vi "EESPY_Read.vi"(2 "I/O Voltage Level":i32(ring)=33 items=["3.3V"=33, "2.5V"=25, "1.8V"=18, "1.5V"=15, "1.2V"=12], 3 "Line Number":u8, 4 "device reference in":T2) -> (0 "Value":bool, 1 "Read Value":T1 items=["0 (Logic Low)", "1 (Logic High)"])   [LabVIEW 2016]
doc: "This basic DIO example uses the DIO basic API to read a digital line. It allows you to change the line number and I/O voltage.\n\nThe parameters will have the following effects:\nLine Number specifies the DIO line to read.\n\nThe I/O Voltage Level property configures the NI-845x reference voltage to the desired level. I/O Voltage Level uses the following values: 3.3V, 2.5V, 1.8V, 1.5V, and 1.2V. The default value of this property is 3.3 V. Not all NI-845x Hardware support all Voltage Levels.\n\nThe DIO Line Direction Map property sets the line direction map for the active DIO Port. The value is a bitmap that specifies the function of each individual line within the port. If bit x = 1, line x is an output. If bit x = 0, line x is an input. The value of this property is set to 0 for the chosen line\n\nFor connection information see the 845x Software User Manual and the manual for your specific device."
uses:
  <vilib>/ni845x/ni845x.llb/ni845xControl.ctl
  <vilib>/ni845x/ni845x.llb/ni845xDioLineWriteValue.ctl
  <vilib>/ni845x/ni845x.llb/NI-845x Close Device Reference.vi
  <resource>/objmgr/NI845x.rc
panel:
  # "Overview: This basic DIO example uses the DIO basic API to read a digital \nline. It allows you to change the line number and I/O voltage.\nRequirements: LabVIEW, NI-XNET\nInstructions:\n1. Select the 845x device you want to use in the device reference in control\n2. Make sure that you've set the I/O Voltage Level appropriately\n3. Run the VI."
  # "(Value is TRUE when Logic High)"
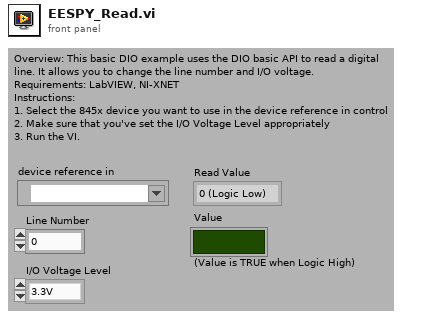
[diagram p1: front panel]
types:
  T1 = typedef "ni845xDioLineWriteValue.ctl" = i32
  T2 = typedef "ni845xControl.ctl" = refnum<k21>
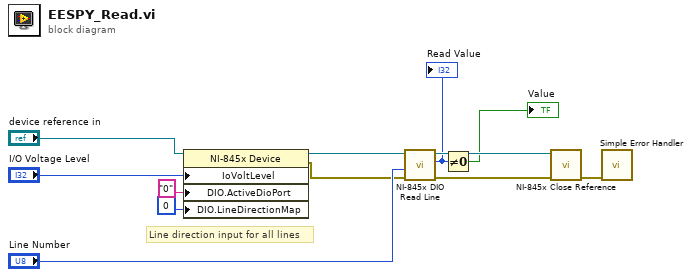
[diagram p0: block diagram]
diagram:
  # "Line direction input for all lines"
  n1 = property class="NI-845x Device"(reference="device reference in", "IoVoltLevel"="I/O Voltage Level", "DIO.ActiveDioPort"="0" ("Active DIO Port"), "DIO.LineDirectionMap"=u8 0 ("DIO Line Direction Map")) -> (reference out=w10:T2, error out=w11:errorcluster)  [unwired: 1 in]
  n2 = call <vilib>:"NI-845x DIO Read Line.vi"("error in (no error)"=w11, "line number (0)"="Line Number", "device reference in"=w10) -> ("error out"=w5:errorcluster, "read value"=w2:T1, "device reference out"=w3:T2)  [unwired: 2 in, 4 out]
  "Read Value" <- w2
  n3 = Not Equal To 0?(x=w2) -> (x != 0?=→"Value":bool)
  n4 = call-poly <vilib>:"NI-845x Close Reference.vi"("error in (no error)"=w5, "device reference"=w3) -> ("error out"=w4:errorcluster)  [unwired: 9 in]
  n5 = call <vilib>:"Simple Error Handler.vi"("error in (no error)"=w4) -> ()  [unwired: 1 in, 8 out]
